vi "ExposeMapperGetContainerTypeFromVariant.vi"(11 "Data Val Ref in":refnum<data-value>) -> (3 "LVPort Labview Contriner type":T1)   [LabVIEW 2017]
uses:
  ExposeObjectMapContainerTypeEnum.ctl
  <vilib>/Utility/Data Type/Type Definitions/Data Type.ctl
  <vilib>/Utility/Data Type/NI_Data Type.lvlib
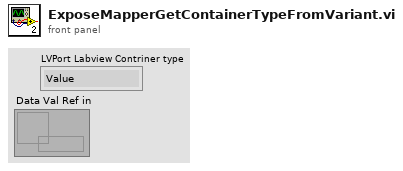
[diagram p1: front panel]
types:
  T1 = typedef "ExposeObjectMapContainerTypeEnum.ctl" = enum16{"Value", "Array", "Waveform", "NetContainer"}
  T2 = typedef "NI_Data Type.lvlib/Data Type.ctl" = enum8{"Invalid Type", "Void", "I8", "I16", "I32", "I64", "U8", "U16", "U32", "U64", "Single Float", "Double Float", "Extended Float", "Single Complex", "Double Complex", "Extended Complex", "Enum U8", "Enum U16", "Enum U32", "Enum U64", "Single Float With Unit", "Double Float With Unit", "Extended Float With Unit", "Single Complex with Unit", "Double Complex with Unit", "Extended Complex with Unit", "Boolean", "String", "Path", "Picture", "Tag", "Array", "Cluster", "Variant", "LV Variant", "Waveform", "Timestamp", "Digital Waveform", "Digital Data", "ExpressData", "Refnum", "External Data", "VI", "Poly VI", "LabVIEW Class Instance", "Fixed Point"}
  T3 = typedef "Waveform Subtype Enum__ogtk.ctl" = enum8{"<Not a Waveform Type>", "0x01", "Analog 16-bit signed", "Analog Double-Precision", "0x04", "Analog Single Precision", "Timestamp", "Digital Data", "Digital Waveform", "Dynamic Data", "Analog Extended-Precision", "Analog 8-bit unsigned", "Analog 16-bit unsigned", "Analog 32-bit unsigned", "Analog 8-bit signed", "Analog 32-bit signed", "Analog Complex Single-Precision", "Analog Complex Double-Precision", "Analog Complex Extended Precision", "Analog 64-bit signed", "Analog 64-bit unsigned"}
  T4 = typedef "NI_Data Type.lvlib/Refnum Type.ctl" = enum16{"NotARefnum", "UnknownRefnum", "Generic", "Datalog", "ByteStream", "Device", "Occurence", "TCPNetConnection", "Auto", "Menu", "Imaq", "Hardware", "DataSocket", "Visa", "IVI", "UDPNetConnection", "Notifier", "Queue", "Irda", "EventReg", "DotNet", "UserEvent", "Callback", "UNUSED_EMPTY_POSITION", "BlueToothNetConnection", "LVObjApp", "LVObjVI", "LVObjUnknown", "GenericClass", "UserDefinedRefnumTag", "DataValue", "RT FIFO", "TDMS File"}
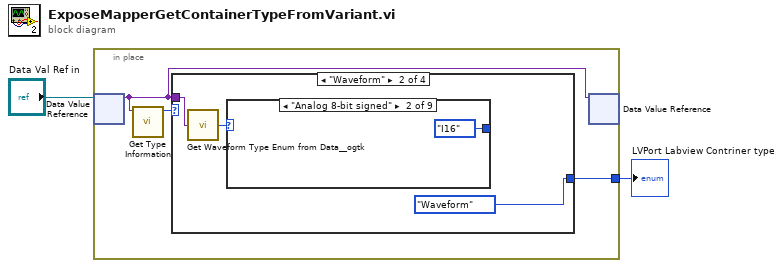
[diagram p0: block diagram]
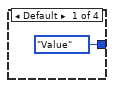
[diagram p2: hidden frame]
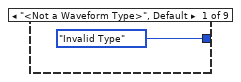
[diagram p3: hidden frame]
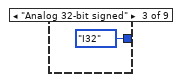
[diagram p4: hidden frame]
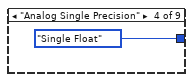
[diagram p5: hidden frame]
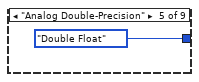
[diagram p6: hidden frame]
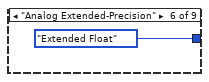
[diagram p7: hidden frame]
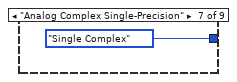
[diagram p8: hidden frame]
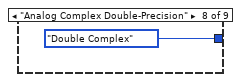
[diagram p9: hidden frame]
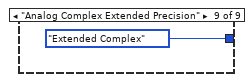
[diagram p10: hidden frame]
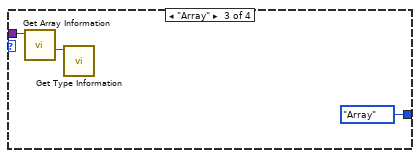
[diagram p11: hidden frame]
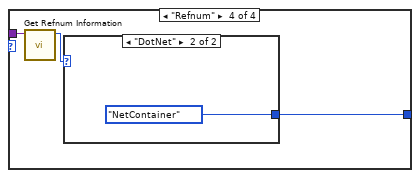
[diagram p12: hidden frame]
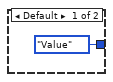
[diagram p13: hidden frame]
diagram:
  n1 = in-place {
    in-place-border: [w4] -> w2
    n2 = in-place-dvr #1("Data Val Ref in") -> (w3:variant)  [unwired: 1 out]
    n3 = call <vilib>:"Get Type Information.vi"("Variant"=w3) -> ("Type"=w5:T2)  [unwired: 6 in, 4 out]
    n4 = case shown="\"Waveform\"" w5 {
      tunnel: w3 -> [_ w9 w21 w24]
      tunnel: [ExposeObjectMapContainerTypeEnum."Value" ExposeObjectMapContainerTypeEnum."Waveform" ExposeObjectMapContainerTypeEnum."Array" w22] -> w4
      frame Default {
      }
      frame "Waveform" {
        n5 = call <userlib>:"Get Waveform Type Enum from Data__ogtk.vi"("Data"=w9) -> ("Waveform Subtype Enum"=w8:T3)  [unwired: 4 in]
        n6 = case shown="\"Analog 8-bit signed\"" w8 {
          tunnel: [Data_Type."Invalid Type" ("Type") Data_Type."I16" ("Type") Data_Type."I32" ("Type") Data_Type."Single Float" ("Type") Data_Type."Double Float" ("Type") Data_Type."Extended Float" ("Type") Data_Type."Single Complex" ("Type") Data_Type."Double Complex" ("Type") Data_Type."Extended Complex" ("Type")] -> _
          frame "<Not a Waveform Type>", Default {
          }
          frame "Analog 8-bit signed" {
          }
          frame "Analog 32-bit signed" {
          }
          frame "Analog Single Precision" {
          }
          frame "Analog Double-Precision" {
          }
          frame "Analog Extended-Precision" {
          }
          frame "Analog Complex Single-Precision" {
          }
          frame "Analog Complex Double-Precision" {
          }
          frame "Analog Complex Extended Precision" {
          }
        }
      }
      frame "Array" {
        n7 = call <vilib>:"Get Array Information.vi"("Variant"=w21) -> ("Array Element Data Type"=w20:variant)  [unwired: 7 in, 3 out]
        n8 = call <vilib>:"Get Type Information.vi"("Variant"=w20) -> ()  [unwired: 6 in, 5 out]
      }
      frame "Refnum" {
        n9 = call <vilib>:"Get Refnum Information.vi"("Variant"=w24) -> ("Reference Type"=w23:T4)  [unwired: 7 in, 3 out]
        n10 = case shown="\"DotNet\"" w23 {
          tunnel: [ExposeObjectMapContainerTypeEnum."Value" ExposeObjectMapContainerTypeEnum."NetContainer"] -> w22
          frame Default {
          }
          frame "DotNet" {
          }
        }
      }
    }
    n11 = in-place-dvr #1(w3) -> ()  [unwired: 2 out]
  }
  "LVPort Labview Contriner type" <- w2
